vi "Handle Type Name.vi"(8 "error in (no error)":errorcluster, 9 "Type":refnum<class>, 10 "JSON":string, 11 "Flatten To JSON Object in":refnum<class "Generic Object Serializer.lvclass">) -> (0 "error out":errorcluster, 1 "Type out":refnum<class>, 2 "JSON out":string, 3 "Flatten To JSON Object out":refnum<class "Generic Object Serializer.lvclass">)   [LabVIEW 2017, in "Generic Object Serializer.lvclass"]
doc: "Extracts type information from a JSON object."
uses:
  Generic Object Serializer/Generic Object Serializer.lvclass
  Generic Object Serializer/Generic Object Serializer.lvclass/Generic Object Serializer.ctl
  Default Serialization Binder/Default Serialization Binder.lvclass
  C:/Users/de200256/Code/logmanoriginal/jsontext-object-serialization/Serialization Binder/Serialization Binder.lvclass
  Serialization Binder/Serialization Binder.lvclass
  <vilib>/JDP Science/JSONtext/JSONtext.lvlib
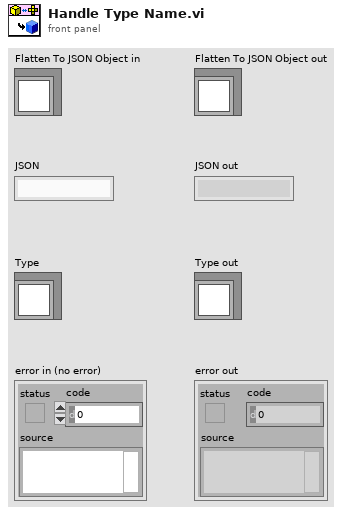
[diagram p1: front panel]
types:
  T1 = typedef "Generic Object Serializer.lvclass/Type Name Handling.ctl" = enum16{"None", "Inline"}
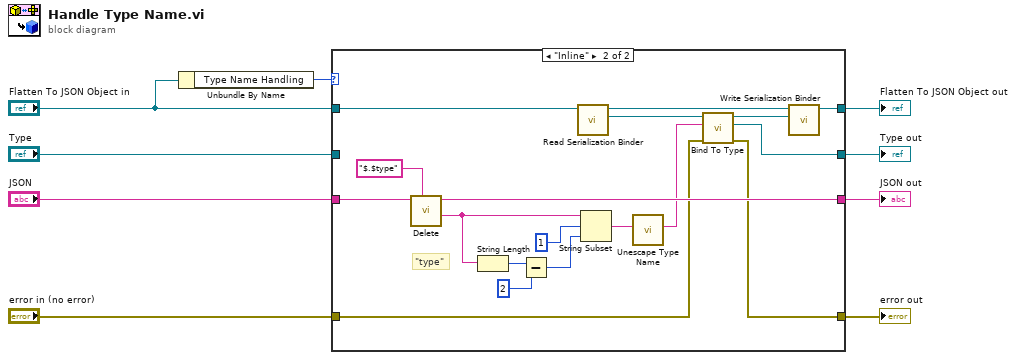
[diagram p0: block diagram]
diagram:
  n1 = Unbundle By Name("Flatten To JSON Object in") -> ("Type Name Handling"=w7:T1)
  n2 = case shown="\"Inline\"" w7 {
    tunnel: "Flatten To JSON Object in" -> [w13 w20]
    tunnel: [w13 w18] -> w8
    tunnel: "JSON" -> [w12 w23]
    tunnel: [w12 w30] -> w5
    tunnel: [w11 w25] -> w4
    tunnel: "Type" -> [w11 _]
    tunnel: "error in (no error)" -> [w10 w22]
    tunnel: [w10 w21] -> w1
    frame Default {
    }
    frame "Inline" {
      # "\"type\""
      n3 = call <vilib>:"Delete.vi"("$Path or Item Name"="$.$type", "JSON"=w23) -> ("<JSON> First Deleted Item"=w24:string, "<JSON>"=w30:string)  [unwired: 5 in, 2 out]
      n4 = String Length(string=w24) -> (length=w28:i32)
      n5 = Subtract(x=w28, y=2) -> (x-y=w26:i32)
      n6 = call "Read Serialization Binder.vi"("Flatten To JSON Object in"=w20) -> ("Serialization Binder"=w17:refnum<class "Serialization Binder.lvclass">, "Flatten To JSON Object out"=w19:refnum<class "Generic Object Serializer.lvclass">)  [unwired: 8 in, 1 out]
      n7 = String Subset(string=w24, offset (0)=1, length (rest)=w26) -> (substring=w15:string)
      n8 = call "Unescape Type Name.vi"("String"=w15) -> ("String out"=w14:string)  [unwired: 10 in]
      n9 = call-dynamic "Bind To Type.vi"("error in (no error)"=w22, "Type Name"=w14, "Serialization Binder in"=w17) -> ("error out"=w21:errorcluster, "Type"=w25:refnum<class>, "Serialization Binder out"=w16:refnum<class "Serialization Binder.lvclass">)  [unwired: 6 in]
      n10 = call "Write Serialization Binder.vi"("Serialization Binder"=w16, "Flatten To JSON Object in"=w19) -> ("Flatten To JSON Object out"=w18:refnum<class "Generic Object Serializer.lvclass">)  [unwired: 8 in, 1 out]
    }
  }
  "error out" <- w1
  "Flatten To JSON Object out" <- w8
  "JSON out" <- w5
  "Type out" <- w4
